vi "Generate Item ID.vi"(11 "Customer DAO In":refnum<class "Object DAO JSON.lvclass">) -> (3 "Customer DAO Out":refnum<class "Object DAO JSON.lvclass">)   [LabVIEW 2020, in "Object DAO JSON.lvclass"]
doc: "Generates an ID for the new Item."
uses:
  Object DAO JSON.lvclass
  C:/Users/fflores/Desktop/DataBase - Copy - Copy/Object DAO/Object DAO.lvclass
  Object DAO/Object DAO.lvclass/Object DAO.ctl
  Object DAO/Member Accessors/Get Object Information.vi
  Object DAO/Member Accessors/Get prefix.vi
  Object DAO/Member Accessors/Set Object Information.vi
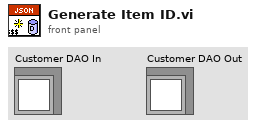
[diagram p1: front panel]
types:
  T1 = typedef "Object DAO.lvclass/Object Information.ctl" = cluster{"String":string, "Boolean":bool, "Numeric":dbl, "id":string}
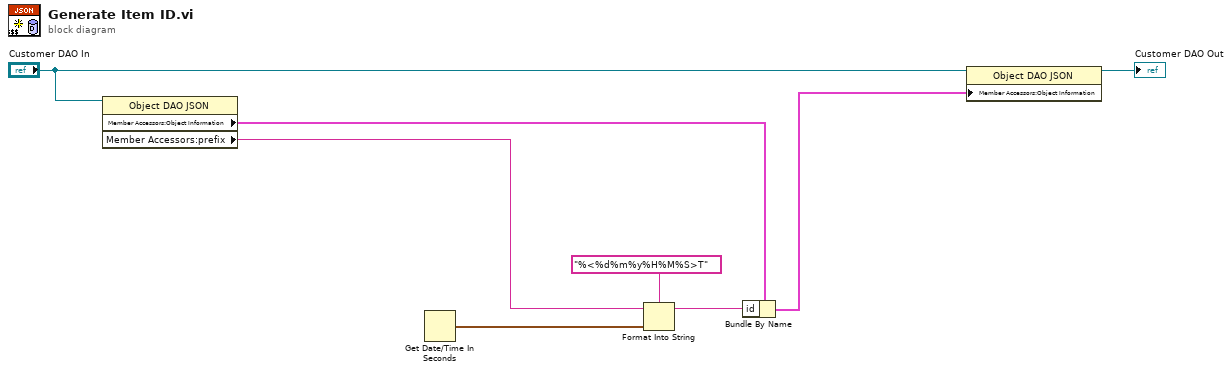
[diagram p0: block diagram]
diagram:
  n1 = property class="Object DAO JSON"(reference="Customer DAO In") -> ("Member Accessors:Object Information"=w5:T1, "Member Accessors:prefix"=w1:string)  [unwired: 1 in, 2 out]
  n2 = Get Date/Time In Seconds() -> (seconds since 1Jan1904=w7:timestamp)
  n3 = Format Into String(format string="%<%d%m%y%H%M%S>T", initial string=w1, w7) -> (resulting string=w6:string)  [unwired: 1 in, 1 out]
  n4 = Bundle By Name(cluster=w5, "id"=w6) -> (w3:T1)
  n5 = property class="Object DAO JSON"(reference="Customer DAO In", "Member Accessors:Object Information"=w3) -> (reference out=→"Customer DAO Out":refnum<class "Object DAO JSON.lvclass">)  [unwired: 1 in, 1 out]
